vi "Create new VIP.vi"(8 "error in (no error)":errorcluster, 10 "String":string="Tooling\\deployment\\Icon editor dev environment.vipb", 11 "Project path":path) -> (0 "error out":errorcluster, 3 "Build Output":path)   [LabVIEW 2021]
uses:
  <vilib>/AppBuilder/AB_API_Simple/NI_App_Builder_API.lvlib
  <vilib>/AppBuilder/AB_API_Simple/Get Build Specification Version (path).vi
  <vilib>/AppBuilder/AB_API_Simple/Build (path).vi
  <vilib>/JKI/VIPM API/VIPM API_vipm_api.lvlib
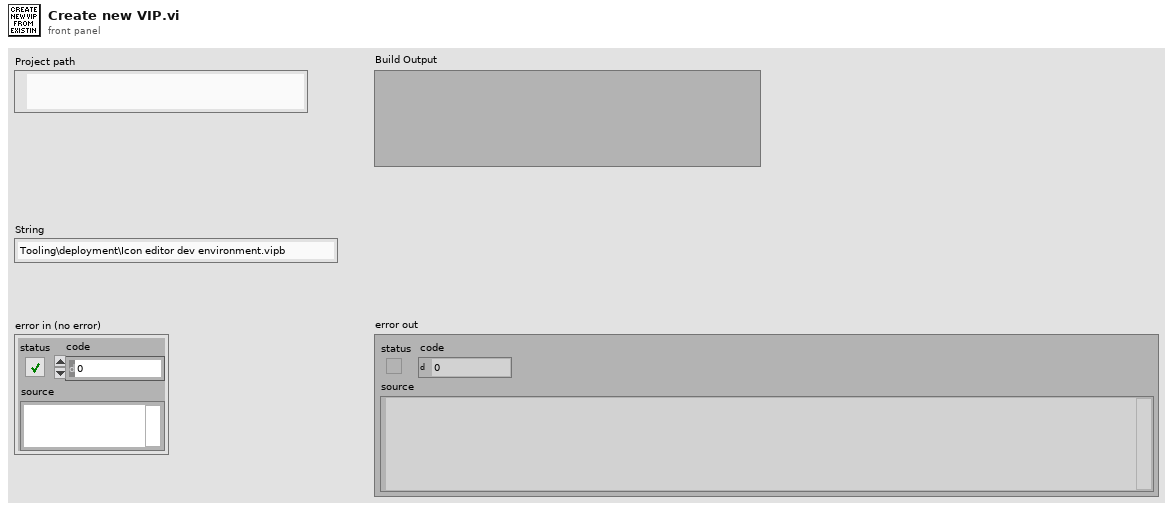
[diagram p1: front panel]
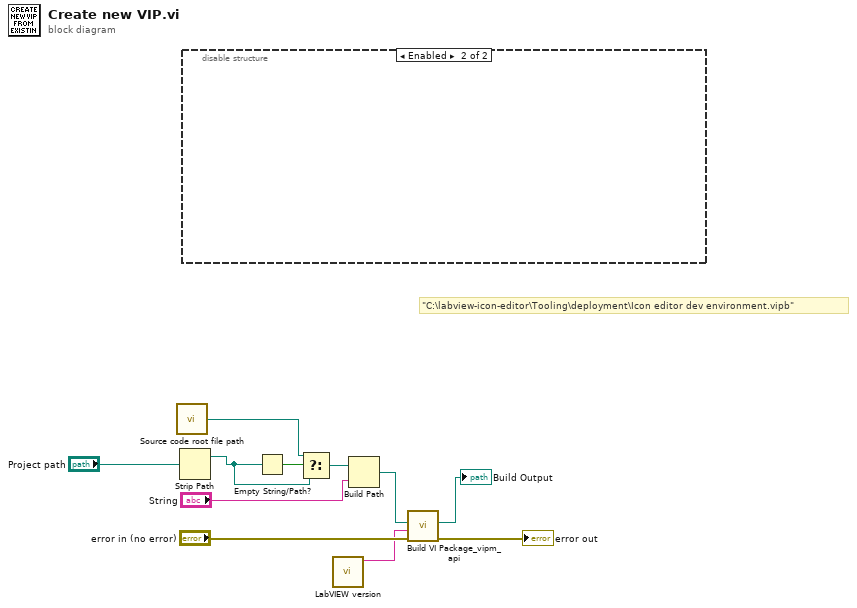
[diagram p0: block diagram]
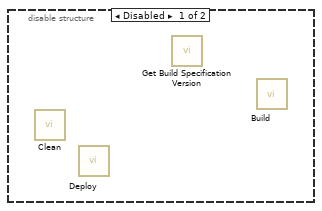
[diagram p2: hidden frame]
diagram:
  # "\"C:\\labview-icon-editor\\Tooling\\deployment\\Icon editor dev environment.vipb\""
  n1 = call "Source code root file path.vi"() -> ("Source code root path"=w10:path)  [unwired: 1 in]
  n2 = Strip Path(path="Project path") -> (stripped path=w1:path)  [unwired: 1 out]
  n3 = disable-structure shown="Enabled" {
    frame Disabled {
      n4 = call <vilib>:"Clean.vi"() -> ()  [unwired: 11 in, 1 out]
      n5 = call <vilib>:"Deploy.vi"() -> ()  [unwired: 11 in, 1 out]
      n6 = call-poly <vilib>:"Get Build Specification Version.vi"() -> ()  [unwired: 10 in, 2 out]
      n7 = call-poly <vilib>:"Build.vi"() -> ()  [unwired: 10 in, 2 out]
    }
    frame Enabled {
    }
  }
  n8 = Empty String/Path?(string/path=w1) -> (empty?=w11:bool)
  n9 = Select(t=w10, s=w11, f=w1) -> (s? t:f=w8:path)
  n10 = call "LabVIEW version.vi"() -> ("Application:Version Year with bitness"=w6:string)  [unwired: 11 in]
  n11 = Build Path(base path=w8, name or relative path="String") -> (appended path=w4:path)
  n12 = call <vilib>:"Build VI Package_vipm_api.vi"("error in (no error)"="error in (no error)", "LabVIEW Version"=w6, "Path to VIPB File"=w4) -> ("error out"=→"error out":errorcluster, "Build Output"=→"Build Output":path)  [unwired: 7 in]
